vi "Get Value.vi"   [LabVIEW 2020, in "CANopen.lvlib" / "Sub Object.lvclass"]
uses:
  Sub Object.lvclass
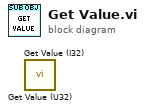
[diagram p0: block diagram]
diagram:
  n1 = call "Get Value (U32).vi"() -> ()  [unwired: 9 in, 3 out]
  n2 = call "Get Value (I32).vi"() -> ()  [unwired: 9 in, 3 out]
